vi "client.vi"() -> ()   [LabVIEW 2010]
panel:
  in  "OK Button":bool
  out "error out":errorcluster
  in  "stop":bool
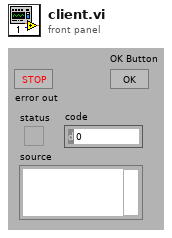
[diagram p1: front panel]
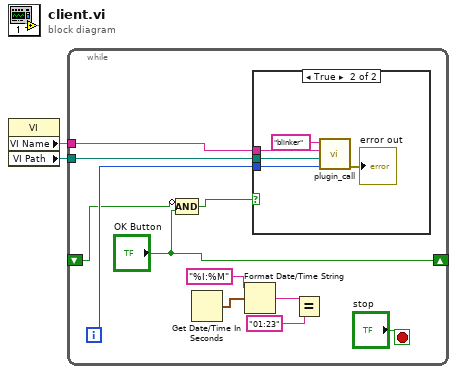
[diagram p0: block diagram]
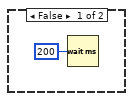
[diagram p2: hidden frame]
diagram:
  n1 = property class="VI"() -> ("VI Name"=w2:string, "VI Path"=w1:path)  [unwired: 2 in, 2 out]
  n2 = while {
    tunnel: w2 -> [w12]
    tunnel: w1 -> [w11]
    shift-right: ["OK Button"] -> _
    shift-left: _ -> [w8]
    i -> [w10]
    stop <- "stop" stop-if-true
    n3 = Compound Arithmetic op=AND(invert w8, "OK Button") -> (w7:bool)
    n4 = Get Date/Time In Seconds() -> (seconds since 1Jan1904=w5:timestamp)
    n5 = Format Date/Time String(time format string (%c)="%I:%M", seconds (now)=w5) -> (date/time string=w4:string)  [unwired: 1 in]
    n6 = case shown="True" w7 {
      tunnel: w12 -> [_ w19]
      tunnel: w11 -> [_ w18]
      tunnel: w10 -> [_ w15]
      frame False {
        n7 = Wait (ms)(milliseconds to wait=u32 200) -> ()  [unwired: 1 out]
      }
      frame True {
        n8 = call "plugin_call.vi"("Data"=w15, "Path"=w18, "Section"=w19, "vi"="blinker") -> ("error out"=→"error out":errorcluster)  [unwired: 3 in]
      }
    }
    n9 = Equal?(x=w4, y="01:23") -> ()  [unwired: 1 out]
  }
